vi "quartering hill climbing.vi"(8 "error in (no error)":errorcluster, 11 "Autofocus in":refnum<class "Autofocus.lvclass">) -> (0 "error out":errorcluster, 3 "Autofocus out":refnum<class "Autofocus.lvclass">)   [LabVIEW 2012, in "Autofocus.lvclass"]
uses:
  Autofocus.lvclass
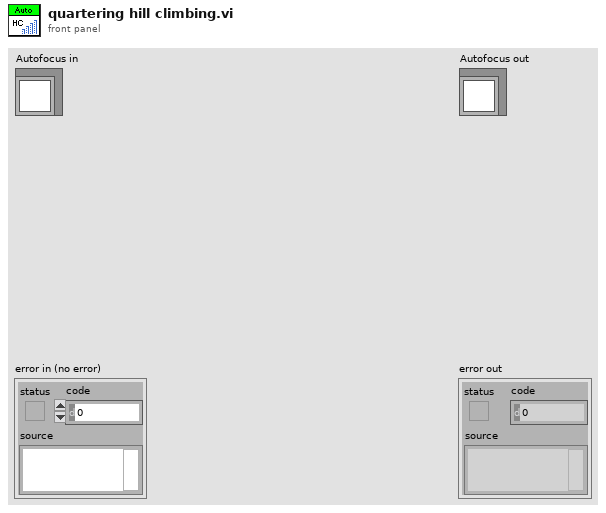
[diagram p1: front panel]
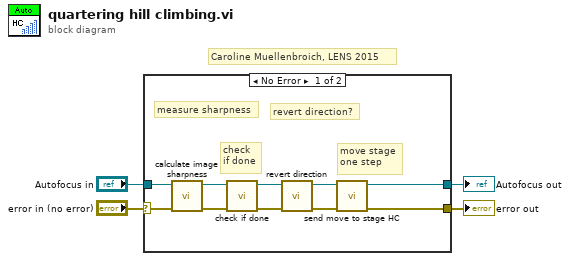
[diagram p0: block diagram]
diagram:
  # "Caroline Muellenbroich, LENS 2015"
  n1 = case shown="No Error" "error in (no error)" {
    selector: "error in (no error)" -> [w14 w16]
    tunnel: [w12 w16] -> w3
    tunnel: [w5 w15] -> w1
    tunnel: "Autofocus in" -> [w6 w15]
    frame No Error {
      # "check\nif done"
      # "move stage\none step"
      # "revert direction?"
      # "measure sharpness"
      n2 = call-dynamic "calculate image sharpness.vi"("error in (no error)"=w14, "Autofocus in"=w6) -> ("error out"=w11:errorcluster, "Autofocus out"=w9:refnum<class "Autofocus.lvclass">)  [unwired: 7 in, 1 out]
      n3 = call-dynamic "check if done.vi"("error in (no error)"=w11, "Autofocus in"=w9) -> ("error out"=w10:errorcluster, "Autofocus out"=w8:refnum<class "Autofocus.lvclass">)  [unwired: 8 in]
      n4 = call-dynamic "revert direction.vi"("error in (no error)"=w10, "Autofocus in"=w8) -> ("error out"=w13:errorcluster, "Autofocus out"=w7:refnum<class "Autofocus.lvclass">)  [unwired: 8 in]
      n5 = call-dynamic "send move to stage HC.vi"("error in (no error)"=w13, "Autofocus in"=w7) -> ("error out"=w12:errorcluster, "Autofocus out"=w5:refnum<class "Autofocus.lvclass">)  [unwired: 8 in]
    }
    frame Error {
    }
  }
  "error out" <- w3
  "Autofocus out" <- w1
